vi "Queue.vi"(0 "Element_In":dbl, 9 "Operation":T1=enum."Enqueue", 11 "Error_In":errorcluster) -> (3 "Overflow":bool, 4 "Element_Out":dbl, 6 "Sum":dbl, 14 "Underflow":bool, 15 "Error_Out":errorcluster)   [LabVIEW 2023]
doc: "This is a LV2, Which has array as its storage unit. hence can be used as queue. it is provided with the pins as follows\nElement_in - Data to be Enqueued\nElement_out - Data Dequeued\nSum - Provides the total sum of elelments in the queue\noverflow and underflow - flags that turns on when overflow and underflow conditions accours.\nError_in and Error_out where given for Error handling"
uses:
  Type_Def/Operation_Queue.ctl
  Type_Def/Size_Pointer.ctl
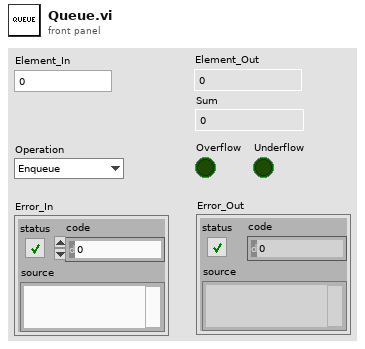
[diagram p1: front panel]
types:
  T1 = typedef "Operation_Queue.ctl" = enum16{"Initialize", "Enqueue", "Dequeue", "Sum"}
  T2 = typedef "Size_Pointer.ctl" = cluster{"Head_Pointer":i64, "Dimension_Size (10)":i64, "Queue":dbl[]}
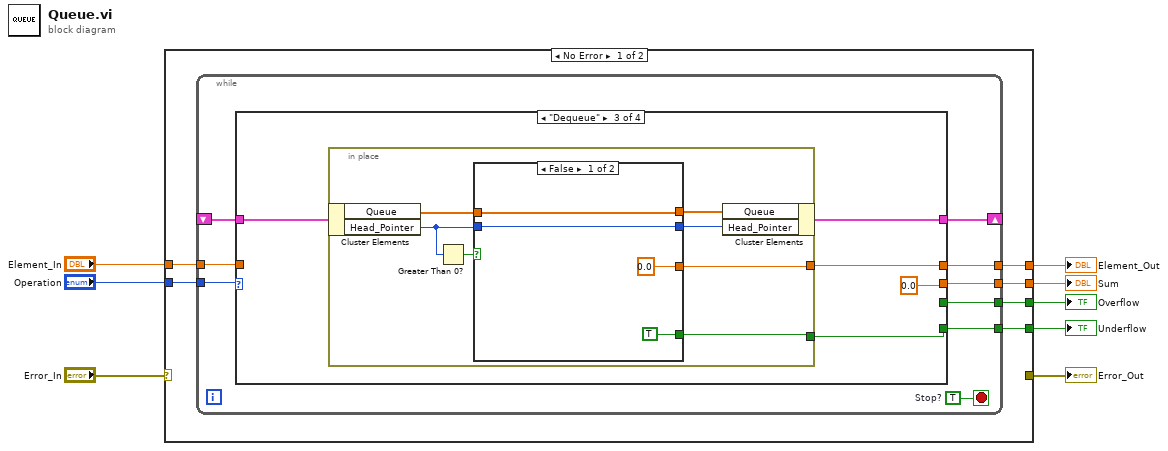
[diagram p0: block diagram]
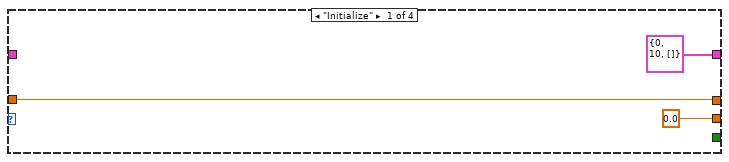
[diagram p2: hidden frame]
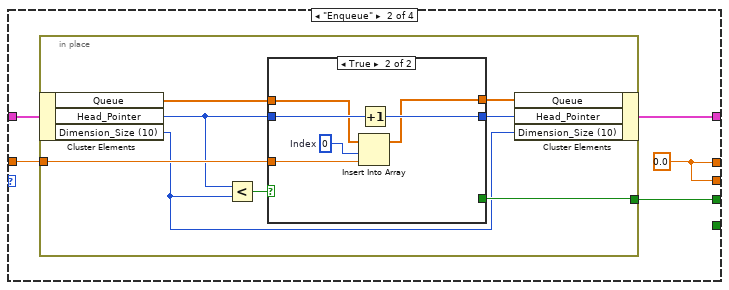
[diagram p3: hidden frame]
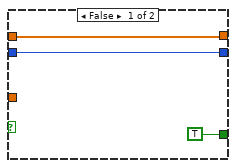
[diagram p4: hidden frame]
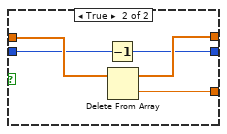
[diagram p5: hidden frame]
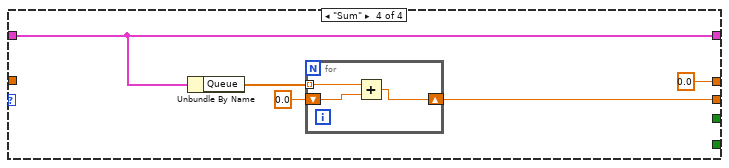
[diagram p6: hidden frame]
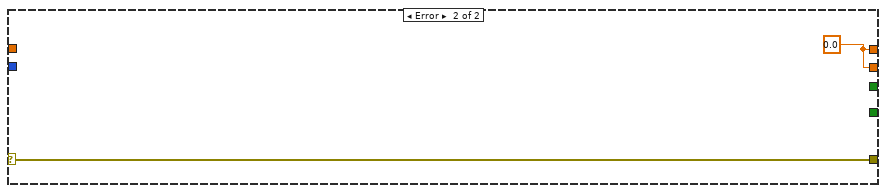
[diagram p7: hidden frame]
diagram:
  n1 = case shown="No Error" "Error_In" {
    selector: "Error_In" -> [_ w79]
    tunnel: [_ w79] -> w7
    tunnel: [w14 w78] -> w6
    tunnel: [w13 w78] -> w5
    tunnel: "Element_In" -> [w12 _]
    tunnel: "Operation" -> [w11 _]
    tunnel: [w10 _] -> w2
    tunnel: [w9 _] -> w1
    frame No Error {
      n2 = while {
        tunnel: [w23] -> w14
        tunnel: [w22] -> w13
        tunnel: w12 -> [w21]
        tunnel: w11 -> [w20]
        tunnel: [w18] -> w10
        tunnel: [w17] -> w9
        shift-right: [w16] -> _
        shift-left: _ -> [w15]
        stop <- w19 stop-if-true
        w19 = TRUE  # Stop?
        n3 = case shown="\"Dequeue\"" w20 {
          tunnel: w15 -> [_ w28 w49 w70]
          tunnel: w21 -> [w25 w31 _ _]
          tunnel: [w25 w29 w53 0.0] -> w23
          tunnel: [0.0 w29 0.0 w73] -> w22
          tunnel: [_ w30 _ _] -> w18
          tunnel: [_ _ w51 _] -> w17
          tunnel: [T2 {"Head_Pointer"=0, "Dimension_Size (10)"=10, "Queue"=[]} ("Queue_and_Pointer") w27 w50 w70] -> w16
          frame "Initialize" {
          }
          frame "Enqueue" {
            w29 = 0.0
            n4 = in-place "In Place Element Structure" {
              in-place-border: w31 -> [w39]
              in-place-border: [w37] -> w30
              n5 = in-place-cluster #1(w28) -> ("Queue"=w36:dbl[], "Head_Pointer"=w33:i64, "Dimension_Size (10)"=w32:i64)
              n6 = Less?(x=w33, y=w32) -> (x < y?=w38:bool)
              n7 = case shown="True" w38 {
                tunnel: w39 -> [_ w45]
                tunnel: w36 -> [w41 w43]
                tunnel: [w41 w46] -> w34
                tunnel: w33 -> [w42 w48]
                tunnel: [w42 w47] -> w35
                tunnel: [TRUE _] -> w37
                frame False {
                }
                frame True {
                  w44 = 0  # Index
                  n8 = Insert Into Array(array=w43, index=w44, new element=w45) -> (w46:dbl[])
                  n9 = Increment(x=w48) -> (x+1=w47:i64)
                }
              }
              n10 = in-place-cluster #1("Queue"=w34, "Head_Pointer"=w35, "Dimension_Size (10)"=w32) -> (w27:T2)
            }
          }
          frame "Dequeue" {
            n11 = in-place "In Place Element Structure" {
              in-place-border: [w60] -> w53
              in-place-border: [w58] -> w51
              n12 = in-place-cluster #2(w49) -> ("Queue"=w55:dbl[], "Head_Pointer"=w56:i64)
              n13 = Greater Than 0?(x=w56) -> (x > 0?=w57:bool)
              n14 = case shown="False" w57 {
                tunnel: [w64 w68] -> w54
                tunnel: w55 -> [w64 w69]
                tunnel: [0.0 w67] -> w60
                tunnel: w56 -> [w63 w66]
                tunnel: [w63 w65] -> w59
                tunnel: [TRUE _] -> w58
                frame False {
                }
                frame True {
                  n15 = Decrement(x=w66) -> (x-1=w65:i64)
                  n16 = Delete From Array(array=w69) -> (deleted portion=w67:dbl, array with subset deleted=w68:dbl[])  [unwired: 2 in]
                }
              }
              n17 = in-place-cluster #2("Queue"=w54, "Head_Pointer"=w59) -> (w50:T2)
            }
          }
          frame "Sum" {
            n18 = Unbundle By Name(w70) -> ("Queue"=w71:dbl[])
            n19 = for {
              tunnel: w71 -> [w77] mode=indexing
              shift-right: [w75] -> w73
              shift-left: 0.0 -> [w76]
              n20 = Add(x=w77, y=w76) -> (x+y=w75:dbl)
            }
          }
        }
      }
    }
    frame Error {
      w78 = 0.0
    }
  }
  "Error_Out" <- w7
  "Element_Out" <- w6
  "Sum" <- w5
  "Overflow" <- w2
  "Underflow" <- w1
